vi "train_GAN_D.vi"(0 "error in (no error)":errorcluster, 1 "ptr":i64, 3 "wasserstein":bool, 4 "Real_fake":bool, 5 "eta":sgl, 7 "lambda":sgl, 8 "gamma":sgl, 9 "buffer array for output":sgl[][](array[numeric]), 11 "last_layer":u32, 12 "input":sgl[][](array[numeric]), 13 "first_layer":u32, 14 "weight_normalization":bool, 15 "RMSprop":bool, 16 "adam":bool, 17 "batch_update":u32, 23 "spectral_norm":bool, 27 "clip":sgl) -> (20 "error out":errorcluster, 21 "ptr out":i64, 24 "critic loss":sgl, 25 "logits":sgl[][](array[numeric]))   [LabVIEW 2016, in "CNet.lvlib"]
uses:
  CNet.lvlib
  Users/jg754/Documents/Visual Studio 2015/Projects/CLearn/x64/Release/CLearn.dll
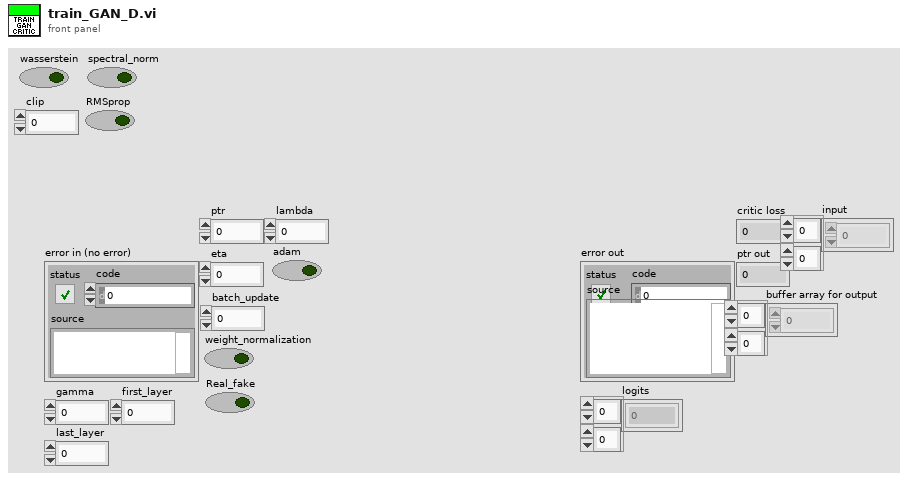
[diagram p1: front panel]
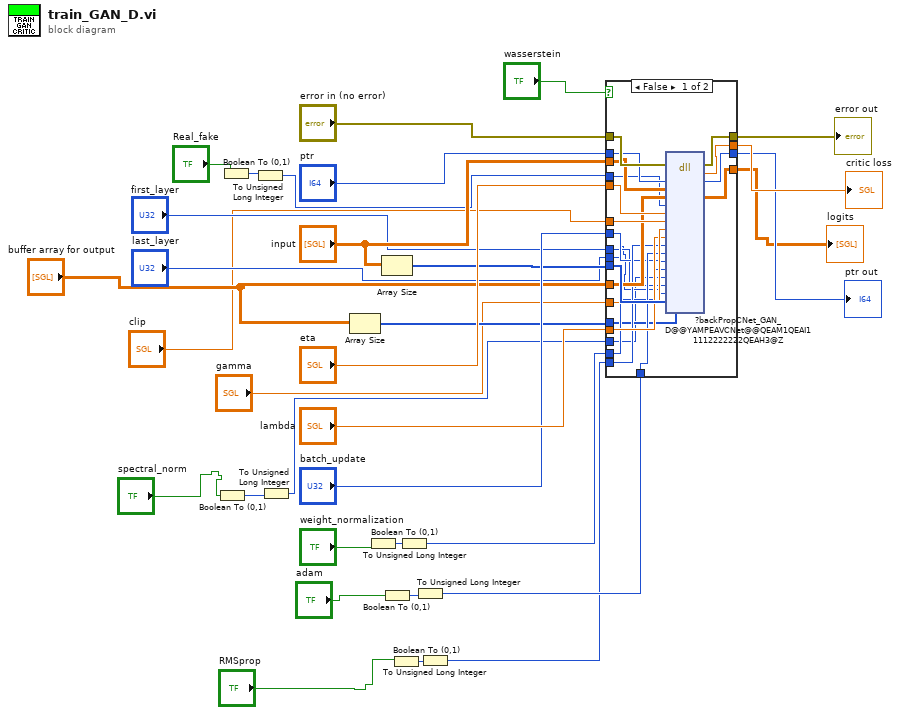
[diagram p0: block diagram]
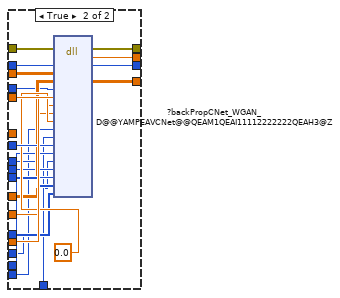
[diagram p2: hidden frame]
diagram:
  n1 = Boolean To (0,1)(Boolean="spectral_norm") -> (0, 1=w4:i16)
  n2 = Boolean To (0,1)(Boolean="Real_fake") -> (0, 1=w14:i16)
  n3 = To Unsigned Long Integer(number=w14) -> (unsigned 32bit integer=w13:u32)
  n4 = To Unsigned Long Integer(number=w4) -> (unsigned 32bit integer=w3:u32)
  n5 = Array Size(array="buffer array for output") -> (size(s)=w19:i32[])
  n6 = Boolean To (0,1)(Boolean="weight_normalization") -> (0, 1=w12:i16)
  n7 = Array Size(array="input") -> (size(s)=w21:i32[])
  n8 = Boolean To (0,1)(Boolean="adam") -> (0, 1=w10:i16)
  n9 = Boolean To (0,1)(Boolean="RMSprop") -> (0, 1=w8:i16)
  n10 = To Unsigned Long Integer(number=w12) -> (unsigned 32bit integer=w11:u32)
  n11 = To Unsigned Long Integer(number=w10) -> (unsigned 32bit integer=w9:u32)
  n12 = To Unsigned Long Integer(number=w8) -> (unsigned 32bit integer=w7:u32)
  n13 = case shown="False" "wasserstein" {
    tunnel: [w54 w77] -> w33
    tunnel: [w43 w76] -> w32
    tunnel: [w52 w75] -> w31
    tunnel: "eta" -> [w50 w74]
    tunnel: "lambda" -> [w45 w73]
    tunnel: "batch_update" -> [w39 w72]
    tunnel: "ptr" -> [w53 w70]
    tunnel: "error in (no error)" -> [w55 w69]
    tunnel: [w44 w68] -> w23
    tunnel: "input" -> [w51 w67]
    tunnel: w21 -> [w48 w66]
    tunnel: "buffer array for output" -> [w47 w65]
    tunnel: w19 -> [w35 w64]
    tunnel: "gamma" -> [w46 w63]
    tunnel: "first_layer" -> [w37 w62]
    tunnel: "last_layer" -> [w36 w61]
    tunnel: w13 -> [w42 w60]
    tunnel: w11 -> [w38 w59]
    tunnel: w9 -> [w40 w58]
    tunnel: w7 -> [w41 w57]
    tunnel: "clip" -> [w49 _]
    tunnel: w3 -> [w34 w56]
    frame False {
      n14 = dll-call lib="C:/Users/jg754/Documents/Visual Studio 2015/Projects/CLearn/x64/Release/CLearn.dll" fn="?backPropCNet_GAN_D@@YAMPEAVCNet@@QEAM1QEAI11112222222QEAH3@Z"(error in=w55, "ptr"=w53, "input"=w51, "outputDesired"=w47, "real"=w42, "eta"=w50, "clip"=w49, "gamma"=w46, "lambda"=w45, "RMSprop"=w41, "adam"=w40, "batch_update"=w39, "weight_normalization"=w38, "spectral_norm"=w34, "first_layer"=w37, "last_layer"=w36, "inFormat"=w48, "outFormat"=w35) -> (error out=w54:errorcluster, "critic_loss"=w43:sgl, "ptr"=w52:i64, "outputDesired"=w44:sgl[][])  [unwired: 17 in, 1 out]
    }
    frame True {
      n15 = dll-call lib="C:/Users/jg754/Documents/Visual Studio 2015/Projects/CLearn/x64/Release/CLearn.dll" fn="?backPropCNet_WGAN_D@@YAMPEAVCNet@@QEAM1QEAI11112222222QEAH3@Z"(error in=w69, "ptr"=w70, "input"=w67, "outputDesired"=w65, "real"=w60, "eta"=w74, "metaEta"=sgl 0.0, "gamma"=w63, "lambda"=w73, "RMSprop"=w57, "adam"=w58, "batch_update"=w72, "weight_normalization"=w59, "spectral_nrom"=w56, "first_layer"=w62, "last_layer"=w61, "inFormat"=w66, "outFormat"=w64) -> (error out=w77:errorcluster, "error"=w76:sgl, "ptr"=w75:i64, "outputDesired"=w68:sgl[][])  [unwired: 17 in, 1 out]
    }
  }
  "error out" <- w33
  "critic loss" <- w32
  "ptr out" <- w31
  "logits" <- w23
